vi "Use Filter Banks in Transmultiplexers.vi"() -> ()   [LabVIEW 2023]
doc: "This example demonstrates how to use filter banks in transmultiplexer applications. Transmultiplexers can convert time-division multiplexed (TDM) signals into frequency-division multiplexed (FDM) signals. This example takes a quadrature amplitude modulated (QAM) signal as the input signal. \nThe synthesis bank converts the input QAM signal into an FDM signal. The analysis bank converts the transmitted FDM signal back to a QAM signal. The received QAM signal is almost the same as the input QAM signal. This example does not take channel C(z) and channel equalizer 1/C(z) into account.\n\nComplete the following steps to use this example:\n1) Run this VI. \n2) On the <b>Transmultiplexer</b> tab, select the <b>Subband Index</b>.\n3) Observe the received signal and the transmitted signal."
uses:
  <vilib>/addons/Digital Filter Design/FilterBank.llb/Process/DFD M-Band Filter Bank Reconstruction (Array).vi
  <vilib>/addons/Digital Filter Design/Process.llb/DFD Integer Delay (Array).vi
  <vilib>/addons/Digital Filter Design/FilterBank.llb/Process/DFD M-Band Filter Bank Decomposition (Array).vi
  <vilib>/addons/Digital Filter Design/NI_DigFilter_FilterBank.lvlib
  <vilib>/addons/Digital Filter Design/NI_DigFilterLicensed.lvlib
panel:
  in  "Tab Control":enum32{"Background", "Transmultiplexer"}(tab)
  out "Real Part":dbl[][](graph)
  in  "Subband Index":u16(ring) items=["Subband 0", "Subband 1", "Subband 2", "Subband 3"]
  out "Image Part":dbl[][](graph)
  in  "stop":bool
  # "Transmultiplexer is one of filter bank applications. Select Help>>Show Context Help and move the cursor over the VI icon of this example for more information."
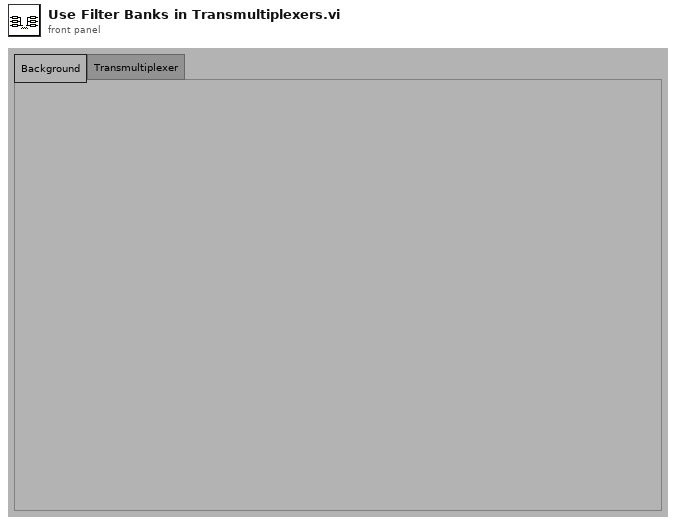
[diagram p1: front panel]
types:
  T1 = typedef "NI_DigFilter_FilterBank.lvlib/DFD Filter Bank Obj.ctl" = cluster{"mFBank_AnalysisFilters":T2[], "mFBank_SynthesisFilters":T2[], "mFBank_#Bands":i32, "mFBank_ProcMethod":T7, "mFBank_Coeffs":dbl[], "mFBank_Gain":dbl, "mFBank_Delay":i32, "mFBank_Type":T8}
  T2 = typedef "NI_DigFilterLicensed.lvlib/DFD Multirate Filter Obj.ctl" = cluster{"mMRate_Structure":enum16{"CIC", "FIR", "IIR", "Lattice"}, "mMRate_Mode":T3, "mMRate_Factor":i32, "mMRate_FIRParams":cluster{"mMRate_FIR_H":dbl[], "mMRate_FIR_IsNyquist?":bool, "mMRate_FIR_IsSymmetric?":bool}, "mMRate_CICParams":cluster{"mMRate_CIC_#Stage":i32, "mMRate_CIC_Lag":i32, "mMRate_CIC_Type":enum16{"Lowpass", "Highpass"}}, "mMRate_Order":i32, "mMRate_Version":string, "mMRate_Comments":string, "mMRate_RationalFactor":cluster{"mMRate_L":i32, "mMRate_M":i32}, "mMRate_Fs":dbl, "mMRate_Quantized?":bool, "mMRate_QFilterGain":dbl, "mMRate_CoefWl":i16, "mMRate_Scaling":cluster{"mMRate_ScaleByPowerOf2?":bool, "mMRate_ScaleType":T4}, "mMRate_InputWl":i16, "mMRate_OutputWl":i16, "mMRate_OutputMode":T5, "mMRate_MultMode":T6, "mMRate_BitPruning":bool, "mMRate_GainWl":i16, "mMRate_OutputFwl":i16, "mMRate_SumIwl":i16, "mMRate_InputIwl ":i16, "mMRate_SumWl":i16, "mMRate_CoefIwl":i16}
  T3 = typedef "NI_DigFilterLicensed.lvlib/DFD Multirate Mode.ctl" = i16
  T4 = typedef "NI_DigFilterLicensed.lvlib/DFD Coef Norm Type.ctl" = enum16{"No Norm", "Time Domain 1-Norm", "Time Domain 2-Norm", "Time Domain Inf-Norm"}
  T5 = typedef "NI_DigFilterLicensed.lvlib/DFD Round-off Mode.ctl" = enum16{"Nearest", "Truncation"}
  T6 = typedef "NI_DigFilterLicensed.lvlib/DFD FXP MRate Multiply Mode.ctl" = enum16{"Truncated", "Full"}
  T7 = typedef "NI_DigFilter_FilterBank.lvlib/DFD Filter Bank Processing Method.ctl" = enum16{"General", "2-Band QMF Lattice", "Cosine-Modulated"}
  T8 = typedef "NI_DigFilter_FilterBank.lvlib/DFD Filter Bank Type.ctl" = u16
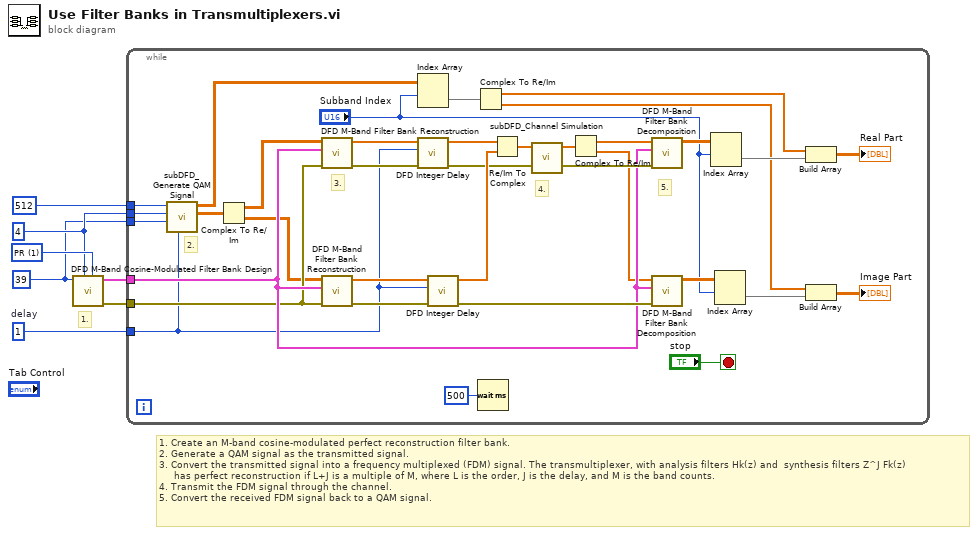
[diagram p0: block diagram]
diagram:
  w7 = u16 1 items=["NPR", "PR"] ("PR?")
  w5 = 4 ("band counts")
  w1 = 39 ("order")
  w2 = 1  # delay
  # "1."
  # "1. Create an M-band cosine-modulated perfect reconstruction filter bank.\n2. Generate a QAM signal as the transmitted signal.\n3. Convert the transmitted signal into a frequency multiplexed (FDM) signal. The transmultiplexer, with analysis filters Hk(z) and  synthesis filters Z^J Fk(z) \n     has perfect reconstruction if L+J is a multiple of M, where L is the order, J is the delay, and M is the band counts.\n4. Transmit the FDM signal through the channel.\n5. Convert the received FDM signal back to a QAM signal."
  n1 = call <vilib>:"DFD M-Band Cosine-Modulated Filter Bank Design.vi"("signal reconstruction"=w7, "band counts"=w5, "order"=w1) -> ("error out"=w3:errorcluster, "filter bank out"=w4:T1)  [unwired: 7 in]
  n2 = while {
    tunnel: 512 -> [w36]
    tunnel: w5 -> [w30]
    tunnel: w4 -> [w22]
    tunnel: w3 -> [w21]
    tunnel: w2 -> [w8]
    tunnel: w1 -> [w12]
    stop <- "stop" stop-if-true
    # "5."
    # "4."
    # "3."
    # "2."
    n3 = call "subDFD_Generate QAM Signal.vi"("delay"=w8, "order"=w12, "#band"=w30, "#signal"=w36) -> ("transmitted signal"=w24:cdb[][], "delayed transmitted signal"=w15:cdb[][])  [unwired: 6 in]
    n4 = Complex To Re/Im(x + iy=w24) -> (x=w20:dbl[][], y=w19:dbl[][])
    n5 = call-poly <vilib>:"DFD M-Band Filter Bank Reconstruction.vi"("error in (no error)"=w21, "filter bank in"=w22, "subband signals"=w20) -> ("error out"=w39:errorcluster, "signal out"=w41:dbl[])  [unwired: 7 in]
    n6 = call-poly <vilib>:"DFD M-Band Filter Bank Reconstruction.vi"("error in (no error)"=w21, "filter bank in"=w22, "subband signals"=w19) -> ("error out"=w38:errorcluster, "signal out"=w40:dbl[])  [unwired: 7 in]
    n7 = Index Array(array=w15, index (row)="Subband Index") -> (element=w28:cdb[])  [unwired: 1 in]
    n8 = call-poly <vilib>:"DFD Integer Delay.vi"("error in (no error)"=w39, "delay"=w8, "signal in"=w41) -> ("error out"=w27:errorcluster, "signal out"=w34:dbl[])  [unwired: 7 in]
    n9 = call-poly <vilib>:"DFD Integer Delay.vi"("error in (no error)"=w38, "delay"=w8, "signal in"=w40) -> ("error out"=w37:errorcluster, "signal out"=w31:dbl[])  [unwired: 7 in]
    n10 = Complex To Re/Im(x + iy=w28) -> (x=w14:dbl[], y=w13:dbl[])
    n11 = Wait (ms)(milliseconds to wait=u32 500) -> ()  [unwired: 1 out]
    n12 = Re/Im To Complex(1:w31, 2:w34) -> (0:w33:cdb[])
    n13 = call "subDFD_Channel Simulation.vi"("transmitted signal"=w33) -> ("recieved signal"=w32:cdb[])  [unwired: 10 out]
    n14 = Complex To Re/Im(x + iy=w32) -> (x=w17:dbl[], y=w18:dbl[])
    n15 = call-poly <vilib>:"DFD M-Band Filter Bank Decomposition.vi"("error in (no error)"=w27, "filter bank in"=w22, "signal in"=w17) -> ("subband signals"=w29:dbl[][])  [unwired: 7 in, 1 out]
    n16 = call-poly <vilib>:"DFD M-Band Filter Bank Decomposition.vi"("error in (no error)"=w37, "filter bank in"=w22, "signal in"=w18) -> ("subband signals"=w26:dbl[][])  [unwired: 7 in, 1 out]
    n17 = Index Array(array=w29, index (row)="Subband Index") -> (element=w35:dbl[])  [unwired: 1 in]
    n18 = Index Array(array=w26, index (row)="Subband Index") -> (element=w16:dbl[])  [unwired: 1 in]
    n19 = Build Array(w14, w35) -> (→"Real Part":dbl[][])
    n20 = Build Array(w13, w16) -> (→"Image Part":dbl[][])
  }
